vi "get column text.vi"(8 "error in":errorcluster, 9 "column types":i32[](array[ring]) items=["INTEGER"=1, "FLOAT"=2, "STRING"=3, "BLOB"=4, "NULL"=5], 10 "column index":i32, 11 "ppStmt":i64) -> (0 "error out":errorcluster, 1 "column types out":i32[](array[ring]) items=["INTEGER"=1, "FLOAT"=2, "STRING"=3, "BLOB"=4, "NULL"=5], 3 "text":string)   [LabVIEW 2014, in "SQLite3LV.lvlib" / "cursor.lvclass"]
uses:
  cursor.lvclass
  msvcrt.dll
  SQLite3LV.lvlib
  sqlite3_64.dll
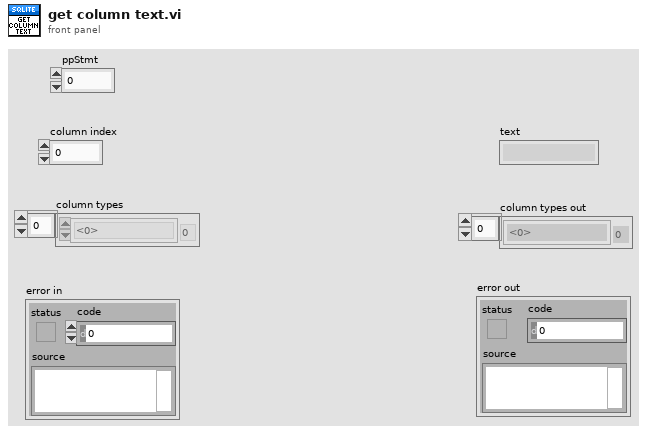
[diagram p1: front panel]
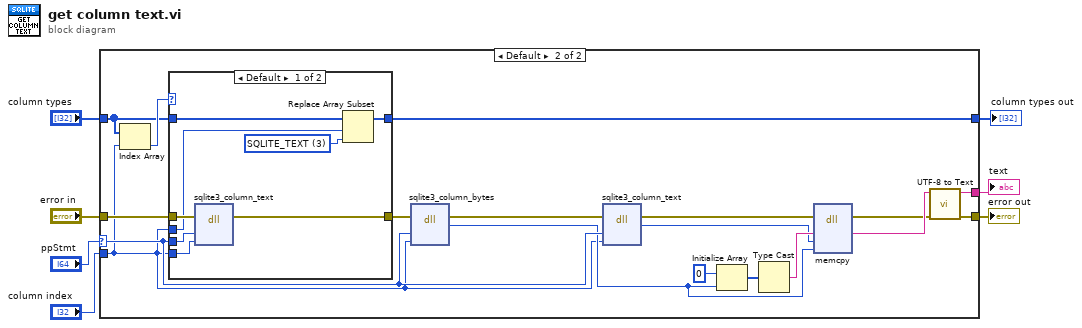
[diagram p0: block diagram]
diagram:
  n1 = case shown="Default" "ppStmt" {
    selector: "ppStmt" -> [_ w20]
    tunnel: [w9 w12] -> w2
    tunnel: "error in" -> [w9 w26]
    tunnel: "column types" -> [w8 w25]
    tunnel: "column index" -> [_ w15]
    tunnel: [_ w13] -> w1
    tunnel: [w8 w10] -> w3
    frame 0 {
    }
    frame Default {
      n2 = Index Array(array=w25, index=w15) -> (element=w27:i32)
      n3 = case shown="Default" w27 {
        tunnel: w26 -> [w35 w37]
        tunnel: [w34 w37] -> w24
        tunnel: w20 -> [w33 _]
        tunnel: w15 -> [w32 _]
        tunnel: w25 -> [w31 w36]
        tunnel: w15 -> [w30 _]
        tunnel: [w28 w36] -> w10
        frame Default {
          w29 = 3 items=["SQLITE_INTEGER"=1, "SQLITE_FLOAT"=2, "SQLITE_TEXT"=3, "SQLITE_BLOB"=4, "SQLITE_NULL"=5] ("new element/subarray")
          n4 = dll-call lib="C:/Users/BobUser/Desktop/LVTables/sqlite3**.*" fn="sqlite3_column_text"(error in=w35, "pStmt"=w33, "iCol"=w32) -> (error out=w34:errorcluster)  [unwired: 5 in, 1 out]
          n5 = Replace Array Subset(array=w31, new element=w29, index=w30) -> (w28:i32[])
        }
        frame 4 {
        }
      }
      n6 = dll-call lib="C:/Users/BobUser/Desktop/LVTables/sqlite3**.*" fn="sqlite3_column_bytes"(error in=w24, "pStmt"=w20, "iCol"=w15) -> (error out=w21:errorcluster, "num bytes"=w19:i32)  [unwired: 4 in, 1 out]
      n7 = dll-call lib="C:/Users/BobUser/Desktop/LVTables/sqlite3**.*" fn="sqlite3_column_text"(error in=w21, "pStmt"=w20, "iCol"=w15) -> (error out=w16:errorcluster, "pChar"=w17:i64)  [unwired: 4 in, 1 out]
      n8 = Initialize Array(u8 0, w19) -> (w22:u8[])
      n9 = Type Cast(x=w22) -> (*(type *) &x=w18:string)  [unwired: 1 in]
      n10 = dll-call lib="msvcrt.dll" fn="memcpy"(error in=w16, "dest"=w18, "src"=w17, "count"=w19) -> (error out=w11:errorcluster, "dest"=w14:string)  [unwired: 5 in, 1 out]
      n11 = call "UTF-8 to Text.vi"("error in"=w11, "utf-8 text"=w14) -> ("error out"=w12:errorcluster, "text"=w13:string)  [unwired: 8 in]
    }
  }
  "column types out" <- w3
  "error out" <- w2
  "text" <- w1
